vi "From String.vi"(8 "error in (no error)":errorcluster, 11 "JSON String":string) -> (0 "error out":errorcluster, 3 "JSON out":refnum<class "JSON Datatype.lvclass">)   [LabVIEW 2015, in "LVJSON.lvlib" / "JSON Datatype.lvclass"]
uses:
  JSON Data Classes/JSON Datatype/JSON Datatype.lvclass
  Token Types.ctl
  <vilib>/Utility/error.llb/whitespace.ctl
  JSON Data Classes/JSON String/New JSON String.vi
  JSON Data Classes/JSON Null/New JSON Null.vi
  JSON Data Classes/JSON Boolean/New JSON Boolean.vi
  JSON Data Classes/JSON Numeric/New JSON Numeric.vi
  JSON Data Classes/JSON Numeric/JSON Numeric.lvclass
  JSON Data Classes/JSON Boolean/JSON Boolean.lvclass
  JSON Data Classes/JSON Null/JSON Null.lvclass
  JSON Data Classes/JSON String/JSON String.lvclass
  JSON Data Classes/JSON Array/JSON Array.lvclass
  JSON Data Classes/JSON Object/JSON Object.lvclass
  LVJSON.lvlib
panel:
  out "Value Tokens":cluster{"Token Type":T1, "Token Value":string}[](array[cluster])
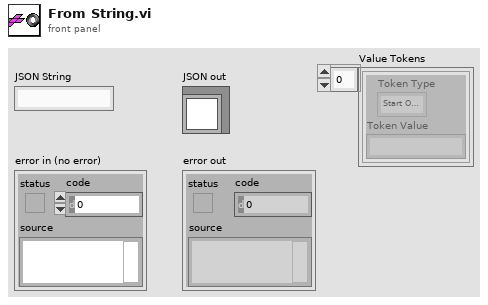
[diagram p1: front panel]
types:
  T1 = typedef "LVJSON.lvlib/Token Types.ctl" = enum32{"Start Object", "End Object", "Start Array", "End Array", "Quotation", "Numeric", "true", "false", "null", "Escape", "Undefined"}
  T2 = typedef "whitespace.ctl" = u16
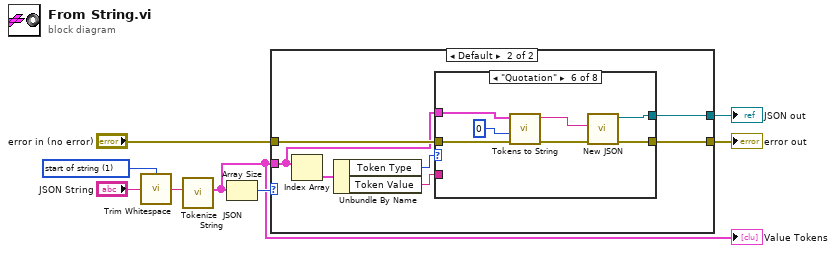
[diagram p0: block diagram]
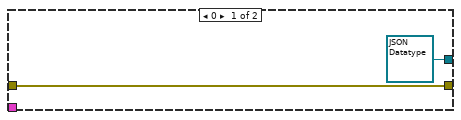
[diagram p2: hidden frame]
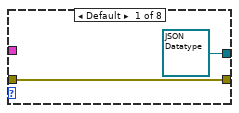
[diagram p3: hidden frame]
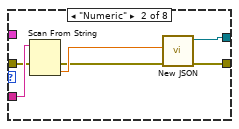
[diagram p4: hidden frame]
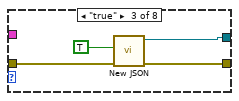
[diagram p5: hidden frame]
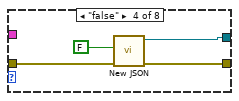
[diagram p6: hidden frame]
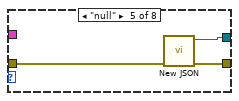
[diagram p7: hidden frame]
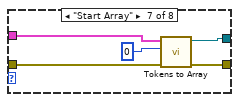
[diagram p8: hidden frame]
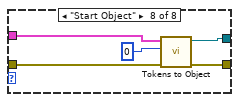
[diagram p9: hidden frame]
diagram:
  w3 = T2 1 items=["both", "start of string", "end of string"] ("location (both)")
  n1 = call <vilib>:"Trim Whitespace.vi"("string"="JSON String", "location (both)"=w3) -> ("trimmed string"=w1:string)
  n2 = call "Tokenize  JSON String.vi"("JSON String"=w1) -> ("Value Tokens"=w7:cluster{"Token Type":T1, "Token Value":string}[])  [unwired: 10 in]
  "Value Tokens" <- w7
  n3 = Array Size(array=w7) -> (size(s)=w8:i32)
  n4 = case shown="Default" w8 {
    tunnel: w7 -> [_ w11]
    tunnel: [refnum<class "JSON Datatype.lvclass"> refnum ("JSON Array out") w14] -> w4
    tunnel: "error in (no error)" -> [w9 w13]
    tunnel: [w9 w12] -> w5
    frame 0 {
    }
    frame Default {
      n5 = Index Array(array=w11) -> (element=w17:cluster{"Token Type":T1, "Token Value":string})  [unwired: 1 in]
      n6 = Unbundle By Name(w17) -> ("Token Type"=w16:T1, "Token Value"=w15:string)
      n7 = case shown="\"Quotation\"" w16 {
        tunnel: w15 -> [_ w25 _ _ _ _ _ _]
        tunnel: [refnum<class "JSON Datatype.lvclass"> refnum ("JSON Array out") w23 w29 w33 w36 w43 w44 w49] -> w14
        tunnel: w13 -> [w18 w22 w27 w31 w35 w38 w46 w51]
        tunnel: [w18 w20 w26 w30 w34 w42 w45 w50] -> w12
        tunnel: w11 -> [_ _ _ _ _ w41 w48 w53]
        frame Default {
        }
        frame "Numeric" {
          n8 = Scan From String(input string=w25, error in=w22) -> (error out=w21:errorcluster, output 1=w24:dbl)  [unwired: 3 in, 2 out]
          n9 = call-poly "New JSON.vi"("error in (no error)"=w21, "value"=w24) -> ("error out"=w20:errorcluster, "JSON String out"=w23:refnum<class "JSON Numeric.lvclass">)  [unwired: 8 in]
        }
        frame "true" {
          n10 = call-poly "New JSON.vi"("error in (no error)"=w27, "value"=TRUE) -> ("error out"=w26:errorcluster, "JSON String out"=w29:refnum<class "JSON Boolean.lvclass">)  [unwired: 8 in]
        }
        frame "false" {
          n11 = call-poly "New JSON.vi"("error in (no error)"=w31, "value"=FALSE) -> ("error out"=w30:errorcluster, "JSON String out"=w33:refnum<class "JSON Boolean.lvclass">)  [unwired: 8 in]
        }
        frame "null" {
          n12 = call-poly "New JSON.vi"("error in (no error)"=w35) -> ("error out"=w34:errorcluster, "JSON String out"=w36:refnum<class "JSON Null.lvclass">)  [unwired: 9 in]
        }
        frame "Quotation" {
          n13 = call "Tokens to String.vi"("error in (no error)"=w38, "start index"=0, "Value Tokens"=w41) -> ("error out"=w37:errorcluster, "String Value"=w39:string)  [unwired: 6 in, 1 out]
          n14 = call-poly "New JSON.vi"("error in (no error)"=w37, "value"=w39) -> ("error out"=w42:errorcluster, "JSON String out"=w43:refnum<class "JSON String.lvclass">)  [unwired: 8 in]
        }
        frame "Start Array" {
          n15 = call "Tokens to Array.vi"("error in"=w46, "starting index"=0, "array w/ subset deleted"=w48) -> ("error out"=w45:errorcluster, "JSON Array out"=w44:refnum<class "JSON Array.lvclass">)  [unwired: 6 in, 1 out]
        }
        frame "Start Object" {
          n16 = call "Tokens to Object.vi"("error in"=w51, "starting index"=0, "array w/ subset deleted"=w53) -> ("error out"=w50:errorcluster, "JSON Object out"=w49:refnum<class "JSON Object.lvclass">)  [unwired: 6 in, 1 out]
        }
      }
    }
  }
  "error out" <- w5
  "JSON out" <- w4
